vi "FindMinSteerAngleError.vi"(2 "Motor Power":dbl format="%#_13g", 3 "Desired Angle":dbl format="%#_13g", 4 "Actual Angle":dbl format="%#_13g") -> (0 "Angle Error":dbl, 1 "Motor Power":dbl)   [LabVIEW 2018]
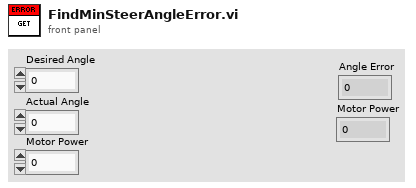
[diagram p1: front panel]
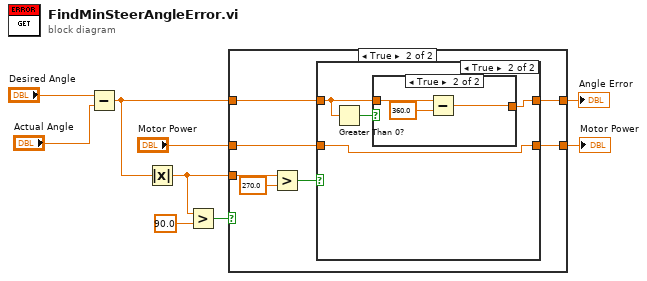
[diagram p0: block diagram]
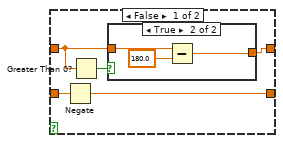
[diagram p3: hidden frame]
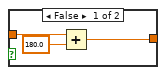
[diagram p4: hidden frame]
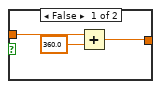
[diagram p5: hidden frame]
diagram:
  n1 = Subtract(x="Desired Angle", y="Actual Angle") -> (x-y=w5:dbl)
  n2 = Absolute Value(x=w5) -> (abs(x)=w3:dbl)
  n3 = Greater?(x=w3, y=90.0) -> (0:w6:bool)
  n4 = case shown="True" w6 {
    tunnel: w5 -> [w10 w16]
    tunnel: "Motor Power" -> [w11 w15]
    tunnel: w3 -> [_ w18]
    tunnel: [w11 w14] -> w2
    tunnel: [w10 w13] -> w1
    frame False {
    }
    frame True {
      n5 = Greater?(x=w18, y=270.0) -> (0:w12:bool)
      n6 = case shown="True" w12 {
        tunnel: w16 -> [w23 w32]
        tunnel: w15 -> [w21 w30]
        tunnel: [w20 w30] -> w14
        tunnel: [w19 w31] -> w13
        frame False {
          n7 = Negate(x=w21) -> (-x=w20:dbl)
          n8 = Greater Than 0?(x=w23) -> (x > 0?=w22:bool)
          n9 = case shown="True" w22 {
            tunnel: w23 -> [w26 w29]
            tunnel: [w24 w27] -> w19
            frame False {
              n10 = Add(x=w26, y=180.0) -> (x+y=w24:dbl)
            }
            frame True {
              n11 = Subtract(x=w29, y=180.0) -> (x-y=w27:dbl)
            }
          }
        }
        frame True {
          n12 = Greater Than 0?(x=w32) -> (x > 0?=w33:bool)
          n13 = case shown="True" w33 {
            tunnel: w32 -> [w36 w39]
            tunnel: [w34 w37] -> w31
            frame False {
              n14 = Add(x=w36, y=360.0) -> (x+y=w34:dbl)
            }
            frame True {
              n15 = Subtract(x=w39, y=360.0) -> (x-y=w37:dbl)
            }
          }
        }
      }
    }
  }
  "Motor Power" <- w2
  "Angle Error" <- w1
